vi "Init.vi"(8 "error in":errorcluster, 10 "args":T4={"ParameterName"="", "Index"=0, "DataType"=0, "DefaultValue"="", "AccessType"=enum."UNKNOWN", "PDOtype"=enum."NO", "Parent"=refnum} {"DataType" items=["UNKNOWN", "BOOLEAN", "INTEGER8", "INTEGER16", "INTEGER32", "UNSIGNED8", "UNSIGNED16", "UNSIGNED32", "REAL32", "VISIBLE_STRING", "OCTET_STRING", "UNICODE_STRING", "TIME_OF_DAY", "TIME_DIFFERENCE", "DOMAIN", "INTEGER24", "REAL64", "INTEGER40", "INTEGER48", "INTEGER56", "INTEGER64", "UNSIGNED24", "UNSIGNED40", "UNSIGNED48", "UNSIGNED56", "UNSIGNED64", "PDO_COMMUNICATION_PARAMETER", "PDO_MAPPING", "SDO_PARAMETER", "IDENTITY"]}, 11 "OD Subentry in":refnum<class "OD Subentry.lvclass">) -> (0 "error out":errorcluster, 3 "OD Subentry out":refnum<class "OD Subentry.lvclass">)   [LabVIEW 2024, in "EDS.lvlib" / "OD Subentry.lvclass"]
uses:
  OD Subentry.lvclass
  OD Subentry.lvclass/OD Subentry.ctl
  Object Type.ctl
  EDS.lvlib
  Data Type.ctl
  Access Type.ctl
  PDO Mapping Type.ctl
  OD Entry/OD Entry.lvclass
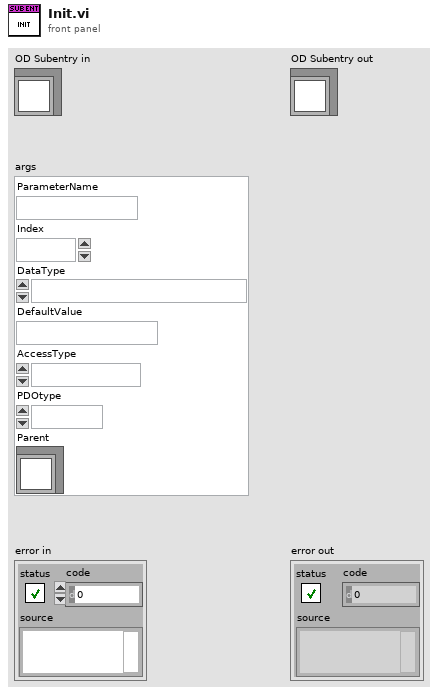
[diagram p1: front panel]
types:
  T1 = typedef "EDS.lvlib/Data Type.ctl" = u16
  T2 = typedef "EDS.lvlib/Access Type.ctl" = enum16{"rw", "ro", "wo", "rwr", "rww", "@const", "UNKNOWN"}
  T3 = typedef "EDS.lvlib/PDO Mapping Type.ctl" = enum16{"NO", "OPTIONAL", "RPDO", "TPDO", "@DEFAULT"}
  T4 = cluster{"ParameterName":string, "Index":u16, "DataType":T1, "DefaultValue":string, "AccessType":T2, "PDOtype":T3, "Parent":refnum<class "OD Entry.lvclass">}
  T5 = typedef "EDS.lvlib/Object Type.ctl" = i16
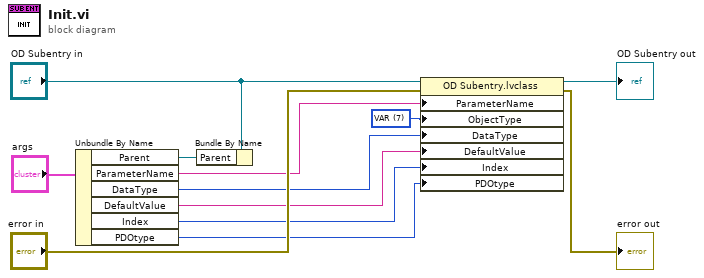
[diagram p0: block diagram]
diagram:
  w5 = T5 7 items=["UNKNOWN"=-1, "NULL"=0, "DOMAIN"=2, "DEFTYPE"=5, "DEFSTRUCT"=6, "VAR"=7, "ARRAY"=8, "RECORD"=9] ("ObjectType")
  n1 = Unbundle By Name("args") -> ("Parent"=w10:refnum<class "OD Entry.lvclass">, "ParameterName"=w6:string, "DataType"=w4:T1, "DefaultValue"=w3:string, "Index"=w2:u16, "PDOtype"=w1:T3)
  n2 = Bundle By Name(cluster="OD Subentry in", "Parent"=w10) -> ()  [unwired: 1 out]
  n3 = property class="OD Subentry.lvclass"(reference="OD Subentry in", error in="error in", "ParameterName"=w6, "ObjectType"=w5, "DataType"=w4, "DefaultValue"=w3, "Index"=w2, "PDOtype"=w1) -> (reference out=→"OD Subentry out":refnum<class "OD Subentry.lvclass">, error out=→"error out":errorcluster)
